vi "arb_2chan.vi"(5 "amp":dbl=0.1 format="%#_13g", 7 "set_amp":bool, 8 "error in (no error)":errorcluster, 9 "wf 2":dbl[](array[numeric]), 10 "wf 1":dbl[](array[numeric]), 11 "device":refnum<visa-resource-name>) -> (0 "error out":errorcluster)   [LabVIEW 2017, in "wf.lvlib"]
uses:
  wf.lvlib
  <vilib>/Instr/_visa.llb/Select Event Type.ctl
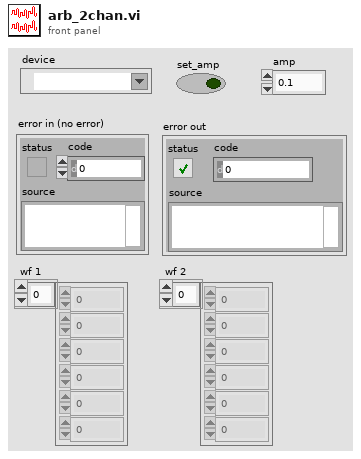
[diagram p1: front panel]
types:
  T1 = typedef "Select Event Type.ctl" = u32
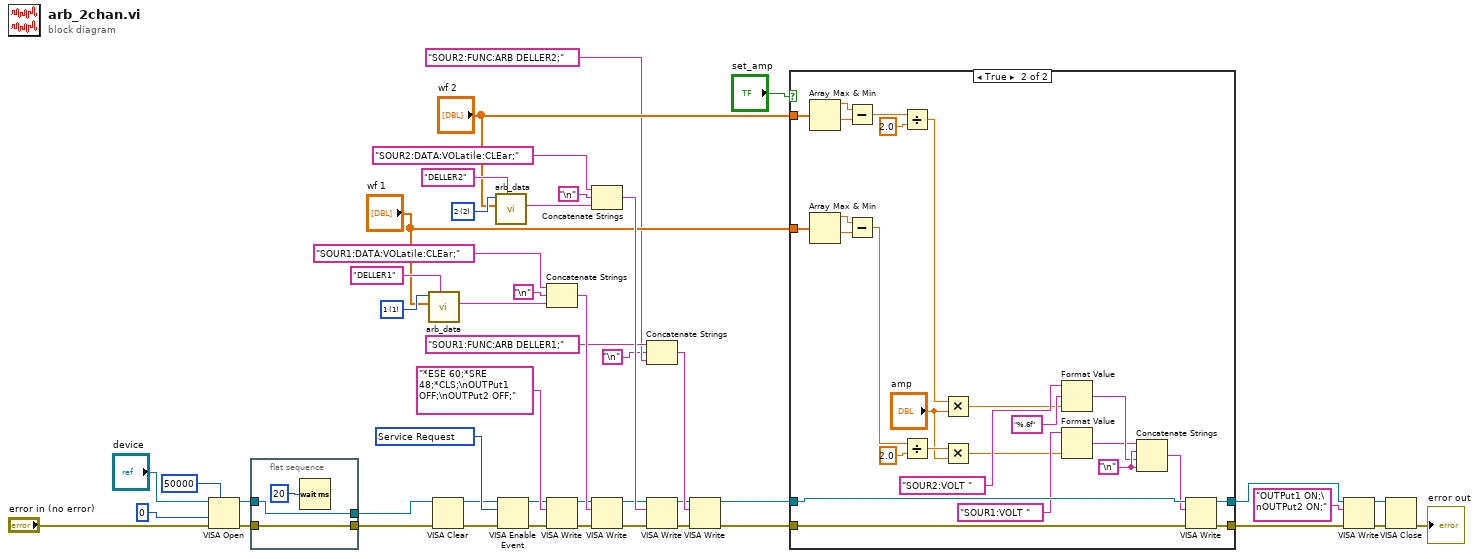
[diagram p0: block diagram]
diagram:
  w31 = 2 items=["1"=1, "2"=2] ("chan")
  w33 = 1 items=["1"=1, "2"=2] ("chan")
  w42 = T1 1073684491 items=["Service Request"=1073684491, "Trigger"=3221168138, "Clear"=1073684493, "VXI Signal"=1073684512, "VXI/VME Interrupt"=3221168161, "VXI/VME Sysfail"=1073684509, "VXI/VME Sysreset"=1073684510, "GPIB CIC"=1073684498, "GPIB Talk"=1073684499, "GPIB Listen"=1073684500, "PXI Interrupt"=1073684514, "Serial Break"=1073684515, "Serial TermChar"=1073684516, "Serial CTS"=1073684521, "Serial DSR"=1073684522, "Serial DCD"=1073684524, "Serial RI"=1073684526, "Serial Character"=1073684533, "USB Interrupt"=1073684535, "All Enabled"=1073709055] ("Event Type")
  n1 = VISA Open(timeout (0)=u32 50000 ("VISA Open timeout (0)"), access mode=u32 0, error in (no error)="error in (no error)", VISA resource name="device") -> (VISA resource name=w45:refnum<visa-resource-name>, error out=w44:errorcluster)  [unwired: 1 out]
  n2 = flat-sequence {
    tunnel: [w49] -> w38
    tunnel: w45 -> [w49]
    tunnel: [w48] -> w39
    tunnel: w44 -> [w48]
    frame #0 {
      n3 = Wait (ms)(milliseconds to wait=u32 20) -> ()  [unwired: 1 out]
    }
  }
  n4 = call "arb_data.vi"("name"="DELLER1", "wf"="wf 1", "chan"=w33) -> ("cmd"=w29:string)  [unwired: 8 in]
  n5 = VISA Clear(VISA resource name=w38, error in (no error)=w39) -> (VISA resource name out=w41:refnum<visa-resource-name>, error out=w40:errorcluster)
  n6 = call "arb_data.vi"("name"="DELLER2", "wf"="wf 2", "chan"=w31) -> ("cmd"=w25:string)  [unwired: 8 in]
  n7 = VISA Enable Event(8:w40, 10:w42, 11:w41) -> (0:w9:errorcluster, 3:w8:refnum<visa-resource-name>)  [unwired: 1 in]
  n8 = Concatenate Strings("SOUR1:DATA:VOLatile:CLEar;", "\n", w29) -> (w27:string)
  n9 = VISA Write(VISA resource name=w8, write buffer="*ESE 60;*SRE 48;*CLS;\nOUTPut1 OFF;\nOUTPut2 OFF;" ("Default Setup String"), error in (no error)=w9) -> (VISA resource name out=w1:refnum<visa-resource-name>, error out=w2:errorcluster)  [unwired: 1 out]
  n10 = Concatenate Strings("SOUR2:DATA:VOLatile:CLEar;", "\n", w25) -> (w23:string)
  n11 = VISA Write(VISA resource name=w1, write buffer=w27, error in (no error)=w2) -> (VISA resource name out=w22:refnum<visa-resource-name>, error out=w21:errorcluster)  [unwired: 1 out]
  n12 = Concatenate Strings("SOUR1:FUNC:ARB DELLER1;", "\n", "SOUR2:FUNC:ARB DELLER2;") -> (w14:string)
  n13 = VISA Write(VISA resource name=w22, write buffer=w23, error in (no error)=w21) -> (VISA resource name out=w11:refnum<visa-resource-name>, error out=w13:errorcluster)  [unwired: 1 out]
  n14 = VISA Write(VISA resource name=w11, write buffer=w14, error in (no error)=w13) -> (VISA resource name out=w10:refnum<visa-resource-name>, error out=w12:errorcluster)  [unwired: 1 out]
  n15 = case shown="True" "set_amp" {
    tunnel: w12 -> [w51 w78]
    tunnel: [w51 w77] -> w6
    tunnel: [w52 w76] -> w7
    tunnel: w10 -> [w52 w75]
    tunnel: "wf 1" -> [_ w63]
    tunnel: "wf 2" -> [_ w58]
    frame False {
    }
    frame True {
      w74 = "\n"
      n16 = Array Max & Min(array=w58) -> (max value=w59:dbl, min value=w60:dbl)  [unwired: 2 out]
      n17 = Array Max & Min(array=w63) -> (max value=w64:dbl, min value=w65:dbl)  [unwired: 2 out]
      n18 = Subtract(x=w59, y=w60) -> (x-y=w61:dbl)
      n19 = Subtract(x=w64, y=w65) -> (x-y=w66:dbl)
      n20 = Divide(x=w61, y=2.0) -> (x/y=w55:dbl)
      n21 = Divide(x=w66, y=2.0) -> (x/y=w57:dbl)
      n22 = Multiply(x=w55, y="amp") -> (x*y=w53:dbl)
      n23 = Multiply(x=w57, y="amp") -> (x*y=w56:dbl)
      n24 = Format Value(string ("")="SOUR2:VOLT ", format string="%.6f", value (0)=w53) -> (output string=w73:string)
      n25 = Format Value(string ("")="SOUR1:VOLT ", value (0)=w56) -> (output string=w72:string)  [unwired: 1 in]
      n26 = Concatenate Strings(w72, w74, w73, w74) -> (w68:string)
      n27 = VISA Write(VISA resource name=w75, write buffer=w68, error in (no error)=w78) -> (VISA resource name out=w76:refnum<visa-resource-name>, error out=w77:errorcluster)  [unwired: 1 out]
    }
  }
  n28 = VISA Write(VISA resource name=w7, write buffer="OUTPut1 ON;\nOUTPut2 ON;" ("Default Setup String"), error in (no error)=w6) -> (VISA resource name out=w5:refnum<visa-resource-name>, error out=w4:errorcluster)  [unwired: 1 out]
  n29 = VISA Close(VISA resource name=w5, error in (no error)=w4) -> (error out=→"error out":errorcluster)
